vi "Snap to Point.vi"(9 "Point":cluster{"x":i32, "y":i32}, 11 "Rect":T1) -> (1 "TopLeft point":cluster{"x":i32, "y":i32}, 3 "Snapped to Point":T1)   [LabVIEW 2012]
doc: "This VI calculates the position of a rectangle that would be centered on the given coordinates (x,y)."
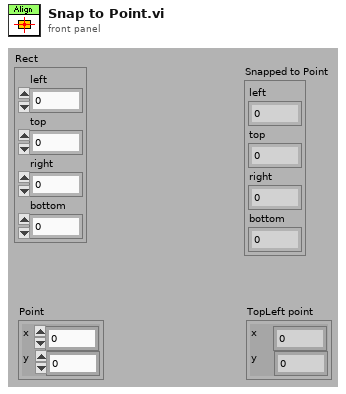
[diagram p1: front panel]
types:
  T1 = cluster{"left":i16, "top":i16, "right":i16, "bottom":i16}
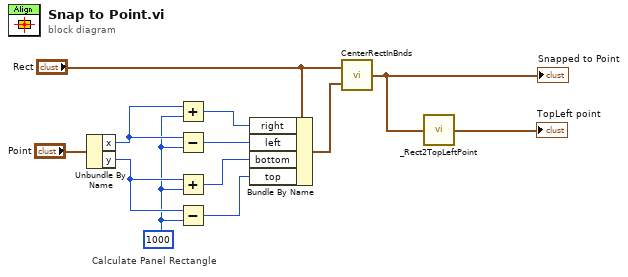
[diagram p0: block diagram]
diagram:
  w7 = 1000 ("x")
  # "Calculate Panel Rectangle"
  n1 = Unbundle By Name("Point") -> ("x"=w9:i32, "y"=w8:i32)
  n2 = Add(x=w9, y=w7) -> (x+y=w4:i32)
  n3 = Subtract(x=w9, y=w7) -> (x-y=w3:i32)
  n4 = Add(x=w8, y=w7) -> (x+y=w2:i32)
  n5 = Subtract(x=w8, y=w7) -> (x-y=w1:i32)
  n6 = Bundle By Name(cluster="Rect", "right"=w4, "left"=w3, "bottom"=w2, "top"=w1) -> (w5:T1)
  n7 = call <vilib>:"CenterRectInBnds.vi"("bounds"=w5, "rect"="Rect") -> ("centered rect"=w12:T1)
  "Snapped to Point" <- w12
  n8 = call "_Rect2TopLeftPoint.vi"("bounds"=w12) -> ("TopLeft point"=→"TopLeft point":cluster{"x":i32, "y":i32})  [unwired: 4 out]
